vi "Create Goals From Last Month.vi"(8 "error in (no error)":errorcluster, 9 "Current Month":T1, 10 "Current YYYY":i32, 11 "Database in":refnum<class "Account History.lvclass">) -> (0 "error out":errorcluster, 3 "Database out":refnum<class "Account History.lvclass">)   [LabVIEW 2018, in "Account History.lvclass"]
uses:
  Account History.lvclass
  Month.ctl
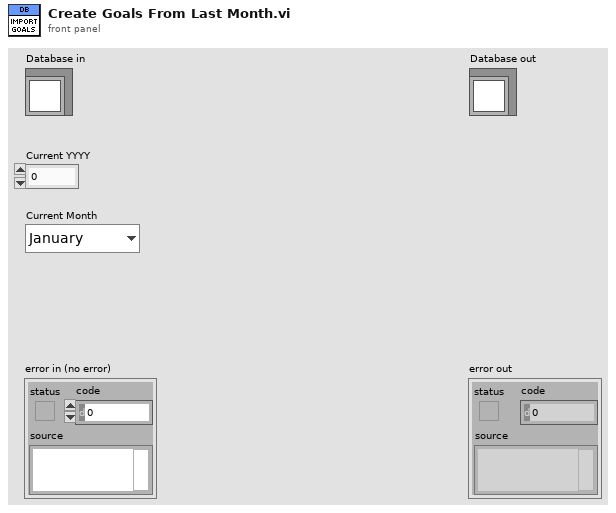
[diagram p1: front panel]
types:
  T1 = typedef "Account History.lvclass/Month.ctl" = enum16{"January", "February", "March", "April", "May", "June", "July", "August", "September", "October", "November", "December"}
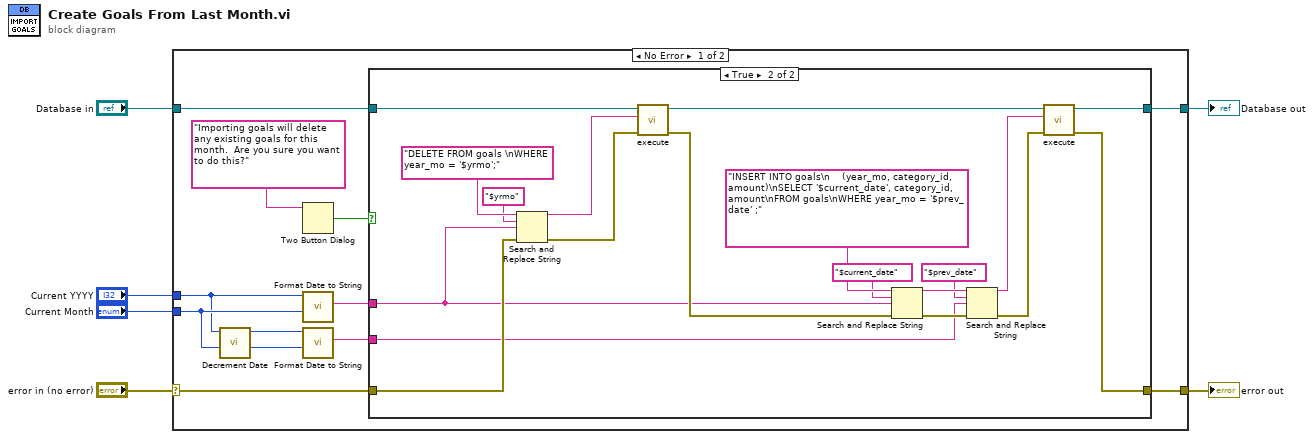
[diagram p0: block diagram]
diagram:
  n1 = case shown="No Error" "error in (no error)" {
    selector: "error in (no error)" -> [w14 w41]
    tunnel: [w13 w41] -> w5
    tunnel: [w15 w40] -> w3
    tunnel: "Database in" -> [w16 w40]
    tunnel: "Current YYYY" -> [w11 _]
    tunnel: "Current Month" -> [w12 _]
    frame No Error {
      n2 = call "Decrement Date.vi"("Current Month"=w12, "Current Year"=w11) -> ("Decremented Month"=w9:T1, "Decremented Year"=w10:i32)  [unwired: 8 in]
      n3 = Two Button Dialog(message="Importing goals will delete any existing goals for this month.  Are you sure you want to do this?") -> (T button?=w17:bool)  [unwired: 2 in]
      n4 = call "Format Date to String.vi"("Month"=w12, "YYYY"=w11) -> ("Year-Mo"=w8:string)  [unwired: 9 in]
      n5 = call "Format Date to String.vi"("Month"=w9, "YYYY"=w10) -> ("Year-Mo"=w7:string)  [unwired: 9 in]
      n6 = case shown="True" w17 {
        tunnel: w16 -> [w20 w36]
        tunnel: [w20 w25] -> w15
        tunnel: w14 -> [w19 w37]
        tunnel: [w19 w24] -> w13
        tunnel: w8 -> [_ w29]
        tunnel: w7 -> [_ w21]
        frame False {
        }
        frame True {
          n7 = Search and Replace String(input string="DELETE FROM goals \nWHERE year_mo = '$yrmo';", search string="$yrmo", replace string=w29, error in=w37) -> (result string=w35:string, error out=w34:errorcluster)  [unwired: 4 in, 2 out]
          n8 = call "execute.vi"("error in (no error)"=w34, "SQL query"=w35, "Database in"=w36) -> ("error out"=w30:errorcluster, "Database out"=w33:refnum<class "Account History.lvclass">)  [unwired: 7 in]
          n9 = Search and Replace String(input string="INSERT INTO goals\n    (year_mo, category_id, amount)\nSELECT '$current_date', category_id, amount\nFROM goals\nWHERE year_mo = '$prev_date' ;", search string="$current_date", replace string=w29, error in=w30) -> (result string=w27:string, error out=w28:errorcluster)  [unwired: 4 in, 2 out]
          n10 = Search and Replace String(input string=w27, search string="$prev_date", replace string=w21, error in=w28) -> (result string=w23:string, error out=w26:errorcluster)  [unwired: 4 in, 2 out]
          n11 = call "execute.vi"("error in (no error)"=w26, "SQL query"=w23, "Database in"=w33) -> ("error out"=w24:errorcluster, "Database out"=w25:refnum<class "Account History.lvclass">)  [unwired: 7 in]
        }
      }
    }
    frame Error {
    }
  }
  "error out" <- w5
  "Database out" <- w3
